vi "OAT Find Equal Values.vi"(1 "array in":i32[](array[numeric])) -> (0 "equal indices":i32[](array[numeric]))   [LabVIEW 2017, in "SoundVib_Gabor.lvlib"]
uses:
  <vilib>/addons/Sound and Vibration/Order Analysis/Gabor Order Tracking/SoundVib_Gabor.lvlib
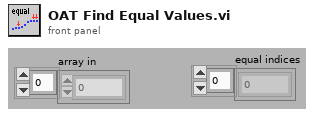
[diagram p1: front panel]
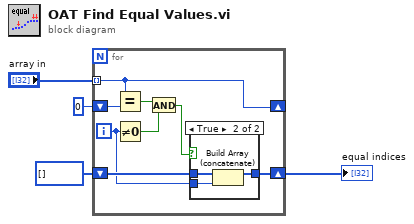
[diagram p0: block diagram]
diagram:
  n1 = for {
    shift-right: [w11] -> _
    shift-left: 0 -> [w12]
    tunnel: "array in" -> [w11] mode=indexing
    shift-right: [w7] -> w4
    shift-left: i32[] [] -> [w6]
    i -> [w5]
    n2 = Equal?(x=w11, y=w12) -> (x = y?=w10:bool)
    n3 = Not Equal To 0?(x=w5) -> (x != 0?=w9:bool)
    n4 = And(x=w10, y=w9) -> (x .and. y?=w8:bool)
    n5 = case shown="True" w8 {
      tunnel: [w13 w16] -> w7
      tunnel: w6 -> [w13 w15]
      tunnel: w5 -> [_ w14]
      frame False {
      }
      frame True {
        n6 = Build Array (concatenate)(w15, w14) -> (w16:i32[])
      }
    }
  }
  "equal indices" <- w4
